vi "uBlaze VIVM.vi"(8 "Control D (+0x000C)":u32 format="%08x", 9 "Control C (+0x0008)":u32 format="%08x", 10 "Control B (+0x0004)":u32 format="%08x", 11 "Control A (+0x0000)":u32 format="%08x") -> (0 "Indicator D (+0x001C)":u32 format="%08x", 1 "Indicator C (+0x0018)":u32 format="%08x", 2 "Indicator B (+0x0014)":u32 format="%08x", 3 "Indicator A (+0x0010)":u32 format="%08x")   [LabVIEW 2011]
uses:
  uBlaze VIVM Globals.vi
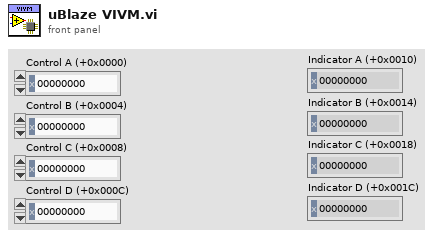
[diagram p1: front panel]
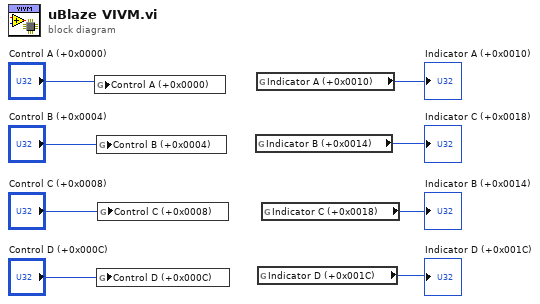
[diagram p0: block diagram]
diagram:
  n1 = global write "uBlaze VIVM Globals.vi" "Control A (+0x0000)"("Control A (+0x0000)") -> ()
  n2 = global write "uBlaze VIVM Globals.vi" "Control B (+0x0004)"("Control B (+0x0004)") -> ()
  n3 = global write "uBlaze VIVM Globals.vi" "Control D (+0x000C)"("Control D (+0x000C)") -> ()
  n4 = global write "uBlaze VIVM Globals.vi" "Control C (+0x0008)"("Control C (+0x0008)") -> ()
  n5 = global read "uBlaze VIVM Globals.vi" "Indicator B (+0x0014)"() -> (→"Indicator C (+0x0018)":u32)
  n6 = global read "uBlaze VIVM Globals.vi" "Indicator A (+0x0010)"() -> (→"Indicator A (+0x0010)":u32)
  n7 = global read "uBlaze VIVM Globals.vi" "Indicator D (+0x001C)"() -> (→"Indicator D (+0x001C)":u32)
  n8 = global read "uBlaze VIVM Globals.vi" "Indicator C (+0x0018)"() -> (→"Indicator B (+0x0014)":u32)
